vi "ReadConfigure__slk_mt.vi"(8 "error in (no error)":errorcluster, 11 "refnum in":T1) -> (0 "error out":errorcluster, 2 "configure values":string[][](array[string]), 3 "refnum out":T1)   [LabVIEW 2013, in "Lazyboots Menu Tool.lvlib"]
doc: "Gets the values from the configure file.\n\n<b>Values:</b>\n[ [Section, Key, Value], [Section, Key, Value], ..., [Section, Key, Value] ]"
uses:
  Library/Lazyboots Menu Tool.lvlib
  <vilib>/Utility/config.llb/NI_LVConfig.lvlib
  <vilib>/Utility/config.llb/Read Key (String).vi
  <vilib>/Utility/config.llb/Config Data RefNum.ctl
panel:
  # "ReadConfigure__slk_mt.vi\nGets the values from the configure file.\n\nNOTICE -- YOU MUST LEAVE THIS NOTICE IN PLACE.\n\nCopyright (c) 2011, LIANG LIU Shawn.Liu.cn@gmail.com\nAll rights reserved.\n\nRedistribution and use in source and binary forms, with or without modification, are permitted provided that the following conditions are met:\n-Redistributions of source code must retain the above copyright notice, this list of conditions and the following disclaimer.\n-Redistributions in binary form must reproduce the above copyright notice, this list of conditions and the following disclaimer in the documentation and/or other materials provided with the distribution.\n-Neither the name of the eLp nor the names of its contributors may be used to endorse or promote products derived from this software without specific prior written permission.\n\nTHIS SOFTWARE IS PROVIDED BY THE COPYRIGHT HOLDERS AND CONTRIBUTORS \"AS IS\" AND ANY EXPRESS OR IMPLIED WARRANTIES, INCLUDING, BUT NOT LIMITED TO, THE IMPLIED WARRANTIES OF MERCHANTABILITY AND FITNESS FOR A PARTICULAR PURPOSE ARE DISCLAIMED. IN NO EVENT SHALL THE COPYRIGHT HOLDER OR CONTRIBUTORS BE LIABLE FOR ANY DIRECT, INDIRECT, INCIDENTAL, SPECIAL, EXEMPLARY, OR CONSEQUENTIAL DAMAGES (INCLUDING, BUT NOT LIMITED TO, PROCUREMENT OF SUBSTITUTE GOODS OR SERVICES; LOSS OF USE, DATA, OR PROFITS; OR BUSINESS INTERRUPTION) HOWEVER CAUSED AND ON ANY THEORY OF LIABILITY, WHETHER IN CONTRACT, STRICT LIABILITY, OR TORT (INCLUDING NEGLIGENCE OR OTHERWISE) ARISING IN ANY WAY OUT OF THE USE OF THIS SOFTWARE, EVEN IF ADVISED OF THE POSSIBILITY OF SUCH DAMAGE."
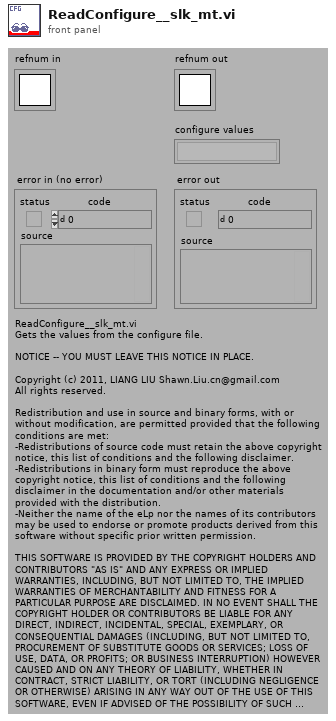
[diagram p1: front panel]
types:
  T1 = typedef "NI_LVConfig.lvlib/Config Data RefNum.ctl" = refnum<k1>
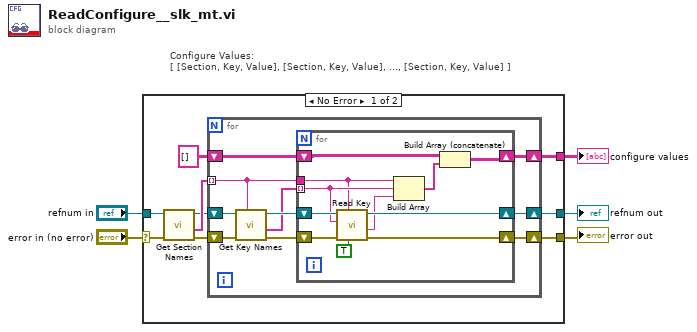
[diagram p0: block diagram]
diagram:
  # "Configure Values:\n[ [Section, Key, Value], [Section, Key, Value], ..., [Section, Key, Value] ]"
  n1 = case shown="No Error" "error in (no error)" {
    selector: "error in (no error)" -> [w9 w36]
    tunnel: "refnum in" -> [w10 w37]
    tunnel: [w8 w36] -> w3
    tunnel: [w7 w37] -> w2
    tunnel: [w6 _] -> w1
    frame No Error {
      n2 = call <vilib>:"Get Section Names.vi"("error in (no error)"=w9, "refnum"=w10) -> ("error out"=w14:errorcluster, "section names"=w13:string[], "refnum out"=w12:T1)  [unwired: 7 out]
      n3 = for {
        tunnel: w13 -> [w18] mode=indexing
        shift-right: [w16] -> w7
        shift-left: w12 -> [w24]
        shift-right: [w15] -> w8
        shift-left: w14 -> [w23]
        shift-right: [w17] -> w6
        shift-left: string[][] [] -> [w19]
        n4 = call <vilib>:"Get Key Names.vi"("section"=w18, "error in (no error)"=w23, "refnum"=w24) -> ("error out"=w21:errorcluster, "key names"=w20:string[], "refnum out"=w22:T1)  [unwired: 6 out]
        n5 = for {
          shift-right: [w32] -> w16
          shift-left: w22 -> [w35]
          shift-right: [w31] -> w15
          shift-left: w21 -> [w34]
          tunnel: w20 -> [w26] mode=indexing
          tunnel: w18 -> [w25]
          shift-right: [w27] -> w17
          shift-left: w19 -> [w29]
          n6 = call-poly <vilib>:"Read Key.vi"("read raw string? (F)"=TRUE, "section"=w25, "error in (no error)"=w34, "key"=w26, "refnum"=w35) -> ("error out"=w31:errorcluster, "value"=w30:string, "refnum out"=w32:T1)  [unwired: 1 in, 3 out]
          n7 = Build Array(w25, w26, w30) -> (w28:string[])
          n8 = Build Array (concatenate)(w29, w28) -> (w27:string[][])
        }
      }
    }
    frame Error {
    }
  }
  "error out" <- w3
  "configure values" <- w1
  "refnum out" <- w2
